vi "Recall Value from TDMS.vi"(6 "Value":variant, 7 "Prefix":string, 8 "Error In":errorcluster, 9 "channel name":string, 10 "group name":string, 11 "tdms file":refnum<k34>) -> (0 "Error Out":errorcluster, 1 "channel name out":string, 2 "group name out":string, 3 "tdms file out":refnum<k34>, 4 "Value out":variant, 5 "found":bool)   [LabVIEW 2016]
uses:
  <vilib>/Utility/Data Type/Type Definitions/Data Type.ctl
  <vilib>/Utility/Data Type/NI_Data Type.lvlib
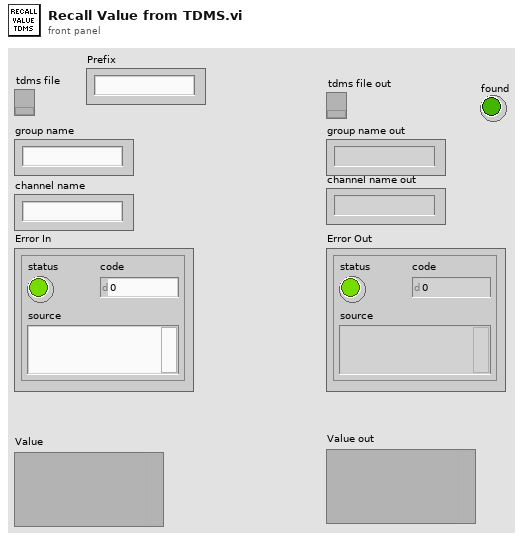
[diagram p1: front panel]
types:
  T1 = typedef "NI_Data Type.lvlib/Data Type.ctl" = enum8{"Invalid Type", "Void", "I8", "I16", "I32", "I64", "U8", "U16", "U32", "U64", "Single Float", "Double Float", "Extended Float", "Single Complex", "Double Complex", "Extended Complex", "Enum U8", "Enum U16", "Enum U32", "Enum U64", "Single Float With Unit", "Double Float With Unit", "Extended Float With Unit", "Single Complex with Unit", "Double Complex with Unit", "Extended Complex with Unit", "Boolean", "String", "Path", "Picture", "Tag", "Array", "Cluster", "Variant", "LV Variant", "Waveform", "Timestamp", "Digital Waveform", "Digital Data", "ExpressData", "Refnum", "External Data", "VI", "Poly VI", "LabVIEW Class Instance", "Fixed Point"}
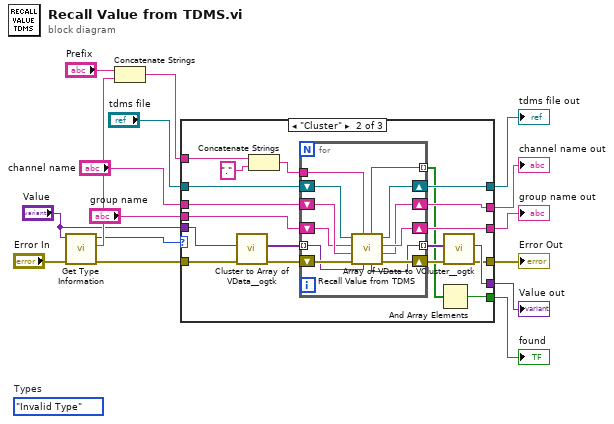
[diagram p0: block diagram]
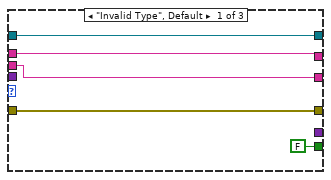
[diagram p2: hidden frame]
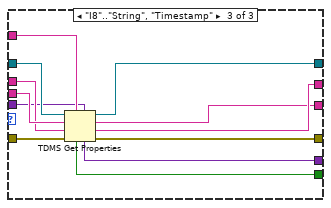
[diagram p3: hidden frame]
diagram:
  (unwired) Data_Type."Invalid Type"  # Types
  n1 = call <vilib>:"Get Type Information.vi"("error in (no error)"="Error In", "Variant"="Value") -> ("error out"=w7:errorcluster, "Name"=w9:string, "Type"=w6:T1)  [unwired: 5 in, 2 out]
  n2 = Concatenate Strings("Prefix", w9) -> (w2:string)
  n3 = case shown="\"Cluster\"" w6 {
    tunnel: "tdms file" -> [w21 w33 w64]
    tunnel: [w21 w32 w63] -> w15
    tunnel: "group name" -> [w19 w24 w62]
    tunnel: "channel name" -> [w18 w25 w61]
    tunnel: [w18 w30 w60] -> w12
    tunnel: [w19 w31 w59] -> w11
    tunnel: w7 -> [w20 w36 w58]
    tunnel: [w20 w27 w57] -> w10
    tunnel: w2 -> [_ w35 w56]
    tunnel: "Value" -> [_ w34 w55]
    tunnel: [FALSE w23 w54] -> w4
    tunnel: [_ w28 w53] -> w3
    frame "Invalid Type", Default {
    }
    frame "Cluster" {
      n4 = call <userlib>:"Cluster to Array of VData__ogtk.vi"("error in (no error)"=w36, "Cluster"=w34) -> ("error out"=w40:errorcluster, "Array of VData"=w39:variant[])  [unwired: 8 in]
      n5 = Concatenate Strings(w35, "." ("string")) -> (w38:string)
      n6 = for {
        shift-right: [w49] -> w26
        shift-left: w40 -> [w51]
        shift-right: [w50] -> w32
        shift-left: w33 -> [w52]
        shift-right: [w44] -> w30
        shift-left: w25 -> [w43]
        shift-right: [w45] -> w31
        shift-left: w24 -> [w42]
        tunnel: w39 -> [w48] mode=indexing
        tunnel: w38 -> [w47]
        tunnel: [w46] -> w29 mode=indexing
        tunnel: [w41] -> w22 mode=indexing
        n7 = call "Recall Value from TDMS.vi"("Value"=w48, "Prefix"=w47, "Error In"=w51, "channel name"=w43, "group name"=w42, "tdms file"=w52) -> ("Error Out"=w49:errorcluster, "channel name out"=w44:string, "group name out"=w45:string, "tdms file out"=w50:refnum<k34>, "Value out"=w46:variant, "found"=w41:bool)
      }
      n8 = And Array Elements(Boolean array=w22) -> (logical AND=w23:bool)
      n9 = call <userlib>:"Array of VData to VCluster__ogtk.vi"("error in (no error)"=w26, "Array"=w29) -> ("error out"=w27:errorcluster, "VCluster"=w28:variant)  [unwired: 8 in]
    }
    frame "I8".."String", "Timestamp" {
      n10 = TDMS Get Properties(5:w55, 7:w56, 8:w58, 9:w61, 10:w62, 11:w64) -> (0:w57:errorcluster, 1:w60:string, 2:w59:string, 3:w63:refnum<k34>, 4:w53:variant, 6:w54:bool)
    }
  }
  "Error Out" <- w10
  "tdms file out" <- w15
  "channel name out" <- w12
  "group name out" <- w11
  "found" <- w4
  "Value out" <- w3
